vi "configure.vi"(8 "error in (no error)":errorcluster, 11 "DL090211FrameImageAssembler in":refnum<class "ImageAssemblerDL090211Frame.lvclass">) -> (0 "error out":errorcluster, 3 "DL090211FrameImageAssembler out":refnum<class "ImageAssemblerDL090211Frame.lvclass">)   [LabVIEW 2010, in "ImageAssemblerDL090211Frame.lvclass"]
uses:
  ImageAssemblerDL090211Frame.lvclass
  ImageAssemblerDL090211Frame.lvclass/ImageAssemblerDL090211Frame.ctl
  common/classes/GenericComponent/GenericComponent/GenericComponent.lvclass
panel:
  in  "bottom cut-off fraction":dbl
  in  "maximum input queue size (data blocks)":i32=-1
  out "Configuration":string
  in  "cancel":bool
  in  "save":bool
  in  "right cut-off fraction":dbl
  in  "left cut-off fraction":dbl
  # "Configure ImageAssemblerDL090211Frame"
  # "Set to -1 for unlimited queue size."
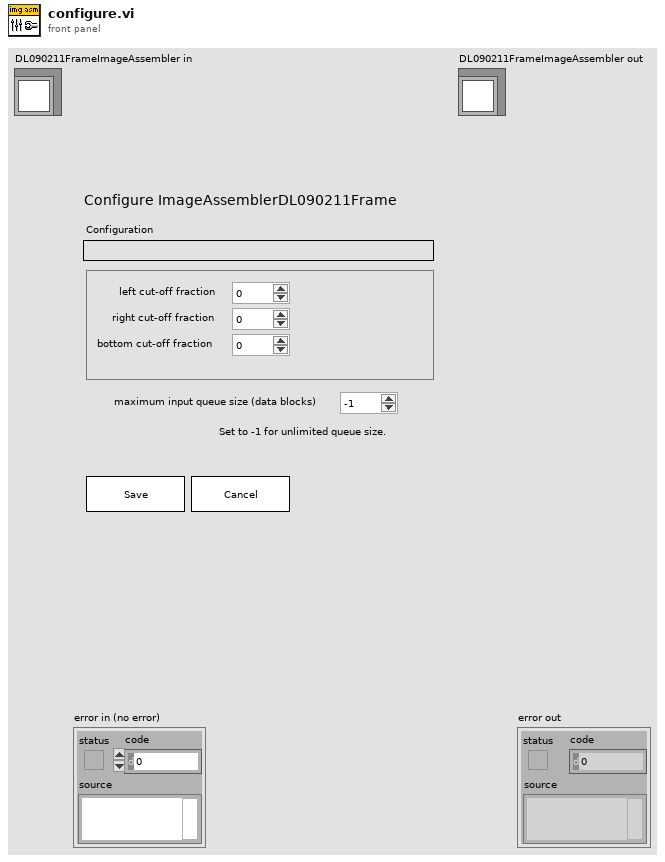
[diagram p1: front panel]
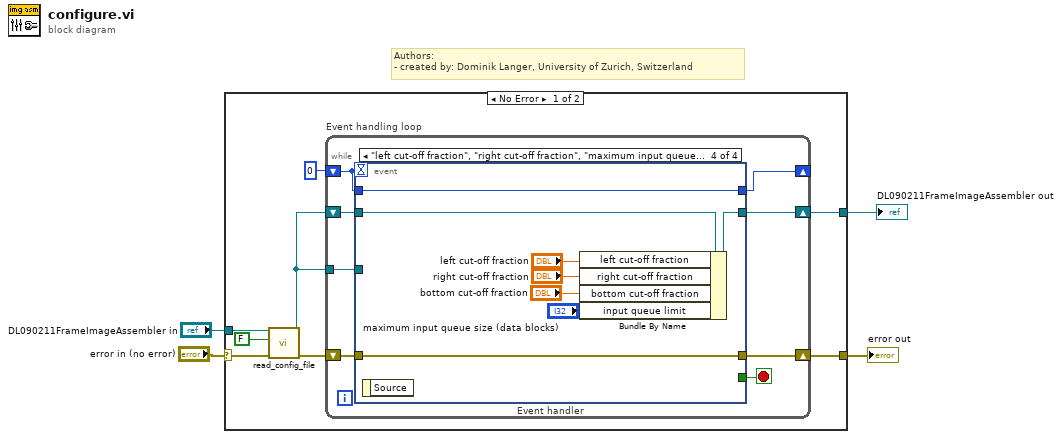
[diagram p0: block diagram]
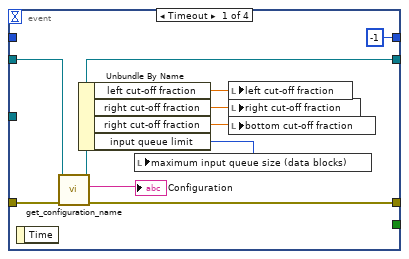
[diagram p2: hidden frame]
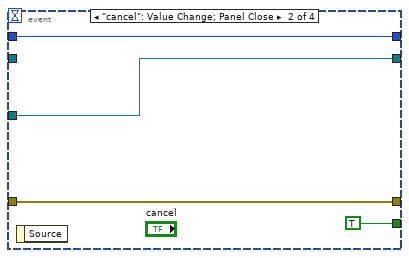
[diagram p3: hidden frame]
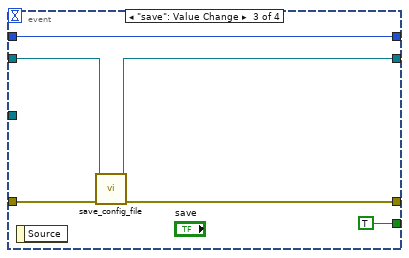
[diagram p4: hidden frame]
diagram:
  # "Authors: \n- created by: Dominik Langer, University of Zurich, Switzerland"
  n1 = case shown="No Error" "error in (no error)" {
    selector: "error in (no error)" -> [w11 w50]
    tunnel: [w8 w50] -> w3
    tunnel: [w6 w49] -> w1
    tunnel: "DL090211FrameImageAssembler in" -> [w10 w49]
    frame No Error {
      n2 = call-dynamic "read_config_file.vi"("error in (no error)"=w11, "force load?"=FALSE, "GenericPlugin in"=w10) -> ("error out"=w9:errorcluster, "GenericPlugin out"=w5:refnum<class "ImageAssemblerDL090211Frame.lvclass">)  [unwired: 7 out]
      n3 = while "Event handling loop" {
        shift-right: [w19] -> w8
        shift-left: w9 -> [w20]
        shift-right: [w17] -> _
        shift-left: 0 -> [w18]
        shift-right: [w14] -> w6
        shift-left: w5 -> [w15]
        tunnel: w5 -> [w13]
        stop <- w16 stop-if-true
        n4 = event "Event handler" shown="[3] \"left cut-off fraction\", \"right cut-off fraction\", \"maximum input queue size (data blocks)\", \"bottom cut-off fraction\": Value Change" {
          selector: _ -> [_ _ _ _]
          dyn-events: _ -> [_ _ _ _]
          timeout: w18 -> [_ _ _ _]
          tunnel: w20 -> [w27 w34 w39 w48]
          tunnel: [w23 w34 w38 w48] -> w19
          tunnel: [-1 w33 w40 w47] -> w17
          tunnel: w18 -> [_ w33 w40 w47]
          tunnel: [_ TRUE TRUE _] -> w16
          tunnel: w15 -> [w26 _ w35 w46]
          tunnel: [w25 w31 w37 w45] -> w14
          tunnel: w13 -> [_ w31 _ _]
          event Timeout {
            n5 = event-data() -> ()  [unwired: 2 out]
            n6 = call "get_configuration_name.vi"("error in (no error)"=w27, "GenericPlugin.lvclass in"=w26) -> ("error out"=w23:errorcluster, "configuration name"=→"Configuration":string, "GenericPlugin.lvclass out"=w25:refnum<class "ImageAssemblerDL090211Frame.lvclass">)  [unwired: 7 in]
            n7 = Unbundle By Name(w25) -> ("left cut-off fraction"=w30:dbl, "right cut-off fraction"=w29:dbl, "right cut-off fraction"=w21:dbl, "input queue limit"=w22:i32)
            n8 = local write "maximum input queue size (data blocks)"(w22) -> ()
            n9 = local write "left cut-off fraction"(w30) -> ()
            n10 = local write "right cut-off fraction"(w29) -> ()
            n11 = local write "bottom cut-off fraction"(w21) -> ()
          }
          event "cancel": Value Change; Panel Close {
            n12 = event-data() -> ()  [unwired: 2 out]
          }
          event "save": Value Change {
            n13 = event-data() -> ()  [unwired: 2 out]
            n14 = call-dynamic "save_config_file.vi"("error in (no error)"=w39, "GenericPlugin in"=w35) -> ("error out"=w38:errorcluster, "GenericPlugin out"=w37:refnum<class "ImageAssemblerDL090211Frame.lvclass">)  [unwired: 2 in, 6 out]
          }
          event "left cut-off fraction", "right cut-off fraction", "maximum input queue size (data blocks)", "bottom cut-off fraction": Value Change {
            n15 = event-data() -> ()  [unwired: 2 out]
            n16 = Bundle By Name(cluster=w46, "left cut-off fraction"="left cut-off fraction", "right cut-off fraction"="right cut-off fraction", "bottom cut-off fraction"="bottom cut-off fraction", "input queue limit"="maximum input queue size (data blocks)") -> (w45:refnum<class "ImageAssemblerDL090211Frame.lvclass">)
          }
        }
      }
    }
    frame Error {
    }
  }
  "error out" <- w3
  "DL090211FrameImageAssembler out" <- w1
